vi "VersaLaseGUI_ForMain_v3.vi"() -> ()   [LabVIEW 2014]
uses:
  D:/Box Sync/Res/LabVIEW/Ts LabVIEW Code/avo/VersaUSB/VersaUSB.dll
  VersaUSB.dll
panel:
  out "Grn Temp 2":dbl
  out "ne":i32
  out "e":i32
  in  "Blu Pow":dbl(slide) scale=0.0..100.0
  in  "Grn Pow":dbl(slide) scale=0.0..40.0
  in  "Blu On":bool
  in  "Grn On":bool
  out "Blu Temp":dbl
  out "Grn Temp":dbl
  in  "Red Pow":dbl(slide) scale=0.0..100.0
  in  "Red On":bool
  out "Red Temp":dbl
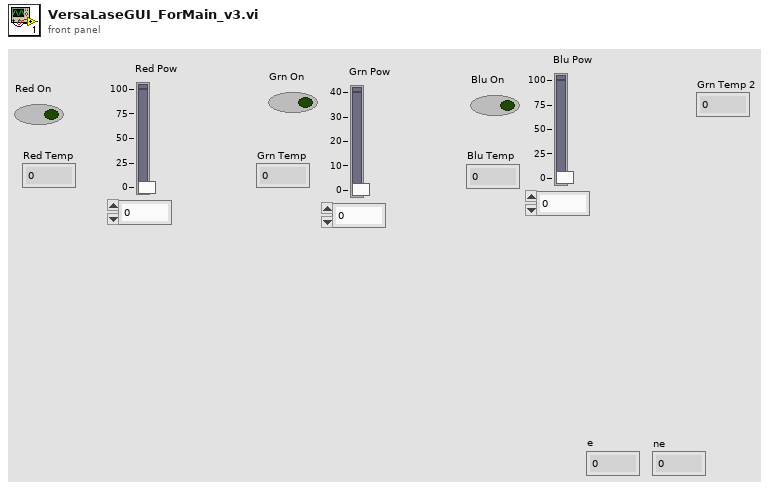
[diagram p1: front panel]
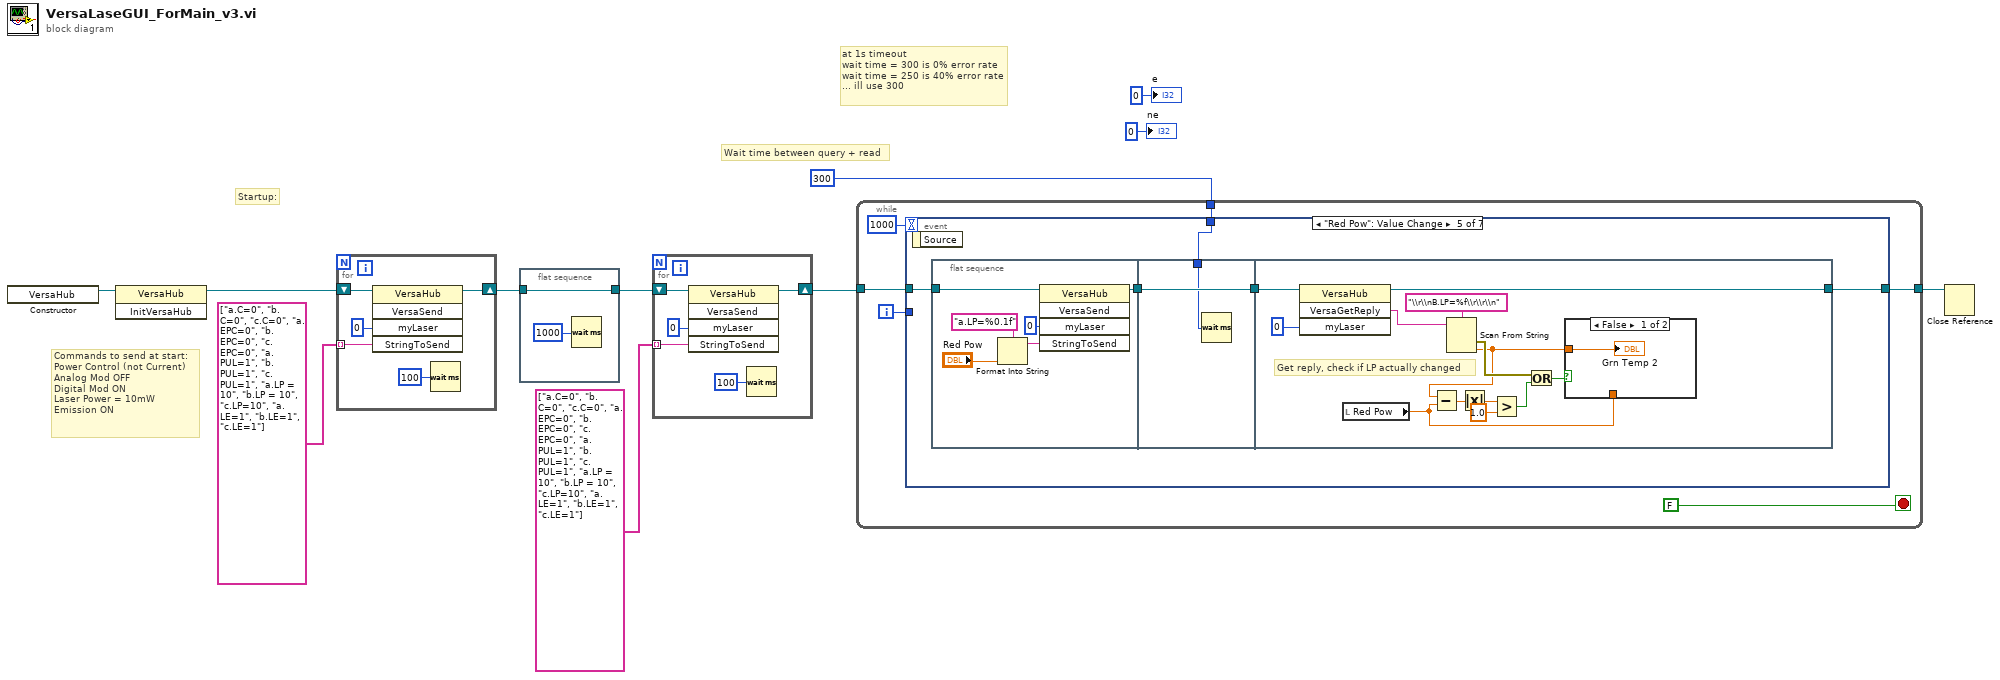
[diagram p0: block diagram]
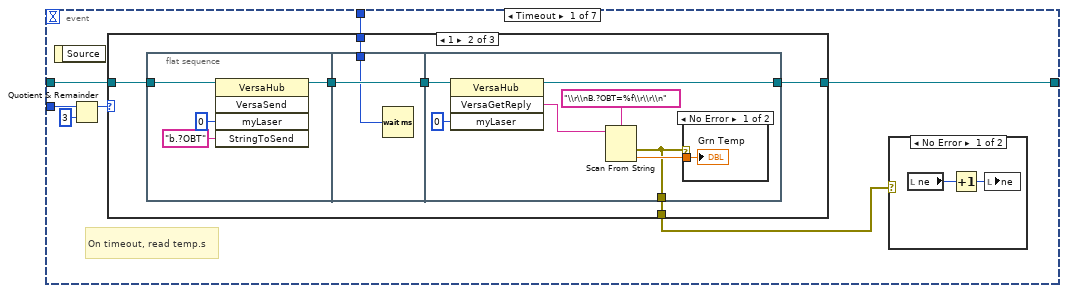
[diagram p2: hidden frame]
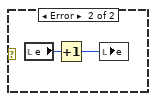
[diagram p3: hidden frame]
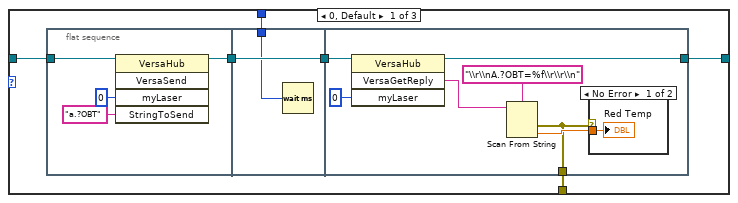
[diagram p4: hidden frame]
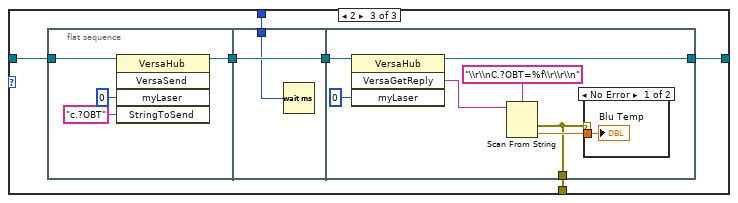
[diagram p7: hidden frame]
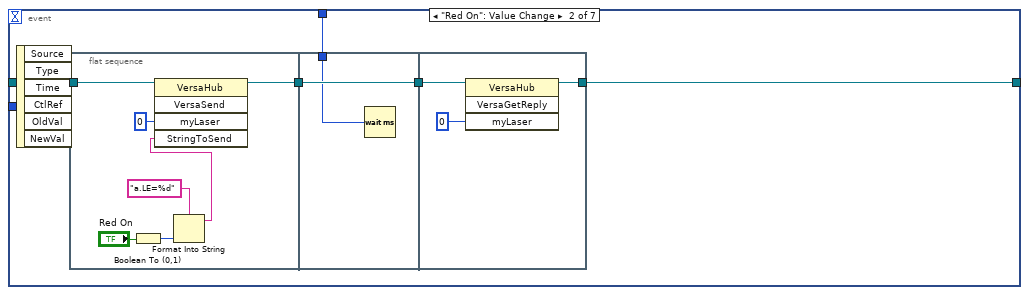
[diagram p9: hidden frame]
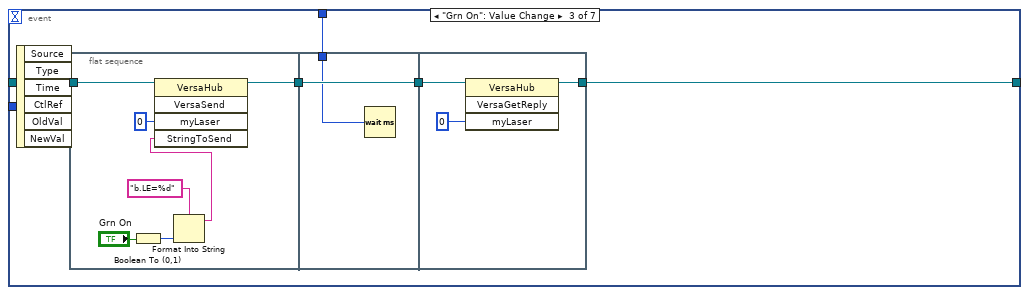
[diagram p10: hidden frame]
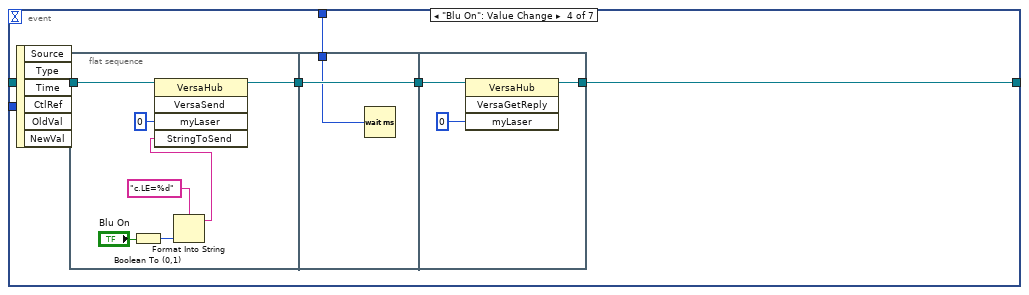
[diagram p11: hidden frame]
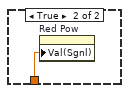
[diagram p12: hidden frame]
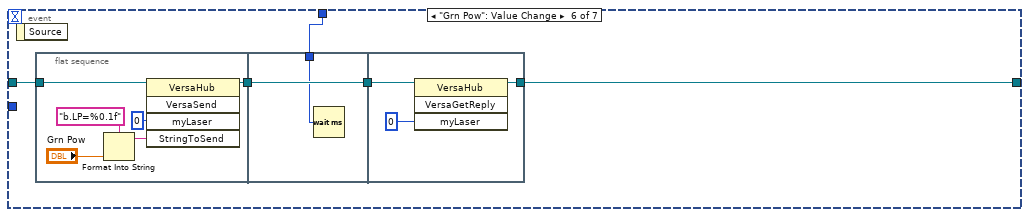
[diagram p13: hidden frame]
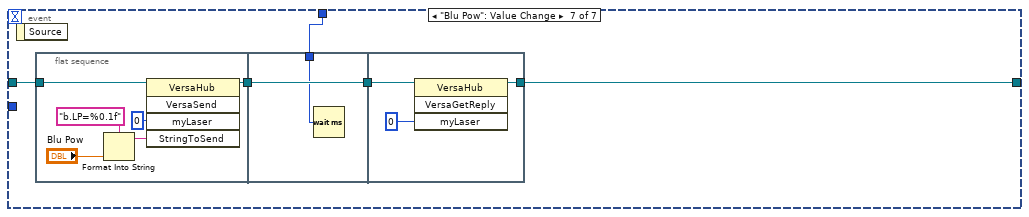
[diagram p14: hidden frame]
diagram:
  # "Startup:"
  # "Wait time between query + read"
  # "Commands to send at start:\nPower Control (not Current)\nAnalog Mod OFF\nDigital Mod ON\nLaser Power = 10mW\nEmission ON"
  # "at 1s timeout\nwait time = 300 is 0% error rate\nwait time = 250 is 40% error rate\n... ill use 300"
  n1 = constructor class="VersaHub"() -> (reference out=w11:refnum<k24>)  [unwired: 3 in, 2 out]
  n2 = invoke class="VersaHub" method="InitVersaHub"(reference=w11) -> (reference out=w5:refnum<k24>)  [unwired: 2 in, 2 out]
  n3 = for {
    tunnel: string[] ["a.C=0", "b.C=0", "c.C=0", "a.EPC=0", "b.EPC=0", "c.EPC=0", "a.PUL=1", "b.PUL=1", "c.PUL=1", "a.LP = 10", "b.LP = 10", "c.LP=10", "a.LE=1", "b.LE=1", "c.LE=1"] -> [w15] mode=indexing
    shift-right: [w14] -> w1
    shift-left: w5 -> [w13]
    n4 = invoke class="VersaHub" method="VersaSend"(reference=w13, "myLaser"=0 ("moduleId"), "StringToSend"=w15) -> (reference out=w14:refnum<k24>)  [unwired: 2 in, 4 out]
    n5 = Wait (ms)(milliseconds to wait=u32 100) -> ()  [unwired: 1 out]
  }
  n6 = flat-sequence {
    tunnel: [w18] -> w2
    tunnel: w1 -> [w18]
    frame #0 {
      n7 = Wait (ms)(milliseconds to wait=u32 1000) -> ()  [unwired: 1 out]
    }
  }
  n8 = for {
    tunnel: string[] ["a.C=0", "b.C=0", "c.C=0", "a.EPC=0", "b.EPC=0", "c.EPC=0", "a.PUL=1", "b.PUL=1", "c.PUL=1", "a.LP = 10", "b.LP = 10", "c.LP=10", "a.LE=1", "b.LE=1", "c.LE=1"] -> [w22] mode=indexing
    shift-right: [w21] -> w3
    shift-left: w2 -> [w20]
    n9 = invoke class="VersaHub" method="VersaSend"(reference=w20, "myLaser"=0 ("moduleId"), "StringToSend"=w22) -> (reference out=w21:refnum<k24>)  [unwired: 2 in, 4 out]
    n10 = Wait (ms)(milliseconds to wait=u32 100) -> ()  [unwired: 1 out]
  }
  n11 = while {
    tunnel: w3 -> [w29]
    tunnel: [w28] -> w10
    tunnel: u32 300 -> [w24]
    i -> [w25]
    stop <- FALSE stop-if-true
    n12 = event shown="[4] \"Red Pow\": Value Change" {
      selector: _ -> [_ _ _ _ _ _ _]
      dyn-events: _ -> [_ _ _ _ _ _ _]
      timeout: 1000 -> [_ _ _ _ _ _ _]
      tunnel: w29 -> [w36 w105 w122 w139 w154 w182 w198]
      tunnel: [w30 w102 w119 w136 w153 w181 w197] -> w28
      tunnel: w25 -> [w35 _ _ _ _ _ _]
      tunnel: w24 -> [w32 w101 w118 w135 w152 w180 w196]
      event Timeout {
        # "On timeout, read temp.s"
        n13 = event-data() -> ()  [unwired: 1 in, 1 out]
        n14 = Quotient & Remainder(x=w35, y=3) -> (x-y*floor(x/y)=w34:i32)  [unwired: 1 out]
        n15 = case shown="1" w34 {
          tunnel: w36 -> [w44 w64 w84]
          tunnel: [w43 w63 w83] -> w30
          tunnel: w32 -> [w42 w62 w82]
          tunnel: [w41 w61 w81] -> w31
          frame 0, Default {
            n16 = flat-sequence {
              tunnel: w44 -> [w50]
              tunnel: [w47] -> w46
              tunnel: w46 -> [w52]
              tunnel: [w52] -> w45
              tunnel: w42 -> [w51]
              tunnel: [w54] -> w43
              tunnel: w45 -> [w58]
              tunnel: [w53] -> w41
              frame #0 {
                n17 = invoke class="VersaHub" method="VersaSend"(reference=w50, "myLaser"=0, "StringToSend"="a.?OBT") -> (reference out=w47:refnum<k24>)  [unwired: 2 in, 4 out]
              }
              frame #1 {
                n18 = Wait (ms)(milliseconds to wait=w51) -> ()  [unwired: 1 out]
              }
              frame #2 {
                n19 = invoke class="VersaHub" method="VersaGetReply"(reference=w58, "myLaser"=0) -> (reference out=w54:refnum<k24>, "VersaGetReply"=w55:string)  [unwired: 2 in, 2 out]
                n20 = Scan From String(format string="\\r\\nA.?OBT=%f\\r\\r\\n", input string=w55) -> (error out=w53:errorcluster, output 1=w56:dbl)  [unwired: 3 in, 2 out]
                n21 = case shown="No Error" w53 {
                  tunnel: w56 -> [w60 _]
                  frame No Error {
                    "Red Temp" <- w60
                  }
                  frame Error {
                  }
                }
              }
            }
          }
          frame 1 {
            n22 = flat-sequence {
              tunnel: w64 -> [w70]
              tunnel: [w67] -> w66
              tunnel: w66 -> [w72]
              tunnel: [w72] -> w65
              tunnel: w62 -> [w71]
              tunnel: [w74] -> w63
              tunnel: w65 -> [w78]
              tunnel: [w73] -> w61
              frame #0 {
                n23 = invoke class="VersaHub" method="VersaSend"(reference=w70, "myLaser"=0, "StringToSend"="b.?OBT") -> (reference out=w67:refnum<k24>)  [unwired: 2 in, 4 out]
              }
              frame #1 {
                n24 = Wait (ms)(milliseconds to wait=w71) -> ()  [unwired: 1 out]
              }
              frame #2 {
                n25 = invoke class="VersaHub" method="VersaGetReply"(reference=w78, "myLaser"=0) -> (reference out=w74:refnum<k24>, "VersaGetReply"=w75:string)  [unwired: 2 in, 2 out]
                n26 = Scan From String(format string="\\r\\nB.?OBT=%f\\r\\r\\n", input string=w75) -> (error out=w73:errorcluster, output 1=w76:dbl)  [unwired: 3 in, 2 out]
                n27 = case shown="No Error" w73 {
                  tunnel: w76 -> [w80 _]
                  frame No Error {
                    "Grn Temp" <- w80
                  }
                  frame Error {
                  }
                }
              }
            }
          }
          frame 2 {
            n28 = flat-sequence {
              tunnel: w84 -> [w90]
              tunnel: [w87] -> w86
              tunnel: w86 -> [w92]
              tunnel: [w92] -> w85
              tunnel: w82 -> [w91]
              tunnel: [w94] -> w83
              tunnel: w85 -> [w98]
              tunnel: [w93] -> w81
              frame #0 {
                n29 = invoke class="VersaHub" method="VersaSend"(reference=w90, "myLaser"=0, "StringToSend"="c.?OBT") -> (reference out=w87:refnum<k24>)  [unwired: 2 in, 4 out]
              }
              frame #1 {
                n30 = Wait (ms)(milliseconds to wait=w91) -> ()  [unwired: 1 out]
              }
              frame #2 {
                n31 = invoke class="VersaHub" method="VersaGetReply"(reference=w98, "myLaser"=0) -> (reference out=w94:refnum<k24>, "VersaGetReply"=w95:string)  [unwired: 2 in, 2 out]
                n32 = Scan From String(format string="\\r\\nC.?OBT=%f\\r\\r\\n", input string=w95) -> (error out=w93:errorcluster, output 1=w96:dbl)  [unwired: 3 in, 2 out]
                n33 = case shown="No Error" w93 {
                  tunnel: w96 -> [w100 _]
                  frame No Error {
                    "Blu Temp" <- w100
                  }
                  frame Error {
                  }
                }
              }
            }
          }
        }
        n34 = case shown="No Error" w31 {
          frame No Error {
            n35 = local read "ne"() -> (w38:i32)
            n36 = Increment(x=w38) -> (x+1=w37:i32)
            n37 = local write "ne"(w37) -> ()
          }
          frame Error {
            n38 = local read "e"() -> (w39:i32)
            n39 = Increment(x=w39) -> (x+1=w40:i32)
            n40 = local write "e"(w40) -> ()
          }
        }
      }
      event "Red On": Value Change {
        n41 = event-data() -> ()  [unwired: 1 in, 6 out]
        n42 = flat-sequence {
          tunnel: w105 -> [w112]
          tunnel: [w110] -> w104
          tunnel: w104 -> [w114]
          tunnel: [w114] -> w103
          tunnel: w101 -> [w113]
          tunnel: [w115] -> w102
          tunnel: w103 -> [w116]
          frame #0 {
            n43 = Boolean To (0,1)(Boolean="Red On") -> (0, 1=w108:i16)
            n44 = Format Into String(format string="a.LE=%d", w108) -> (resulting string=w106:string)  [unwired: 2 in, 1 out]
            n45 = invoke class="VersaHub" method="VersaSend"(reference=w112, "myLaser"=0, "StringToSend"=w106) -> (reference out=w110:refnum<k24>)  [unwired: 2 in, 4 out]
          }
          frame #1 {
            n46 = Wait (ms)(milliseconds to wait=w113) -> ()  [unwired: 1 out]
          }
          frame #2 {
            n47 = invoke class="VersaHub" method="VersaGetReply"(reference=w116, "myLaser"=0) -> (reference out=w115:refnum<k24>)  [unwired: 2 in, 3 out]
          }
        }
      }
      event "Grn On": Value Change {
        n48 = event-data() -> ()  [unwired: 1 in, 6 out]
        n49 = flat-sequence {
          tunnel: w122 -> [w129]
          tunnel: [w127] -> w121
          tunnel: w121 -> [w131]
          tunnel: [w131] -> w120
          tunnel: w118 -> [w130]
          tunnel: [w132] -> w119
          tunnel: w120 -> [w133]
          frame #0 {
            n50 = Boolean To (0,1)(Boolean="Grn On") -> (0, 1=w125:i16)
            n51 = Format Into String(format string="b.LE=%d", w125) -> (resulting string=w123:string)  [unwired: 2 in, 1 out]
            n52 = invoke class="VersaHub" method="VersaSend"(reference=w129, "myLaser"=0, "StringToSend"=w123) -> (reference out=w127:refnum<k24>)  [unwired: 2 in, 4 out]
          }
          frame #1 {
            n53 = Wait (ms)(milliseconds to wait=w130) -> ()  [unwired: 1 out]
          }
          frame #2 {
            n54 = invoke class="VersaHub" method="VersaGetReply"(reference=w133, "myLaser"=0) -> (reference out=w132:refnum<k24>)  [unwired: 2 in, 3 out]
          }
        }
      }
      event "Blu On": Value Change {
        n55 = event-data() -> ()  [unwired: 1 in, 6 out]
        n56 = flat-sequence {
          tunnel: w139 -> [w146]
          tunnel: [w144] -> w138
          tunnel: w138 -> [w148]
          tunnel: [w148] -> w137
          tunnel: w135 -> [w147]
          tunnel: [w149] -> w136
          tunnel: w137 -> [w150]
          frame #0 {
            n57 = Boolean To (0,1)(Boolean="Blu On") -> (0, 1=w142:i16)
            n58 = Format Into String(format string="c.LE=%d", w142) -> (resulting string=w140:string)  [unwired: 2 in, 1 out]
            n59 = invoke class="VersaHub" method="VersaSend"(reference=w146, "myLaser"=0, "StringToSend"=w140) -> (reference out=w144:refnum<k24>)  [unwired: 2 in, 4 out]
          }
          frame #1 {
            n60 = Wait (ms)(milliseconds to wait=w147) -> ()  [unwired: 1 out]
          }
          frame #2 {
            n61 = invoke class="VersaHub" method="VersaGetReply"(reference=w150, "myLaser"=0) -> (reference out=w149:refnum<k24>)  [unwired: 2 in, 3 out]
          }
        }
      }
      event "Red Pow": Value Change {
        n62 = event-data() -> ()  [unwired: 1 in, 1 out]
        n63 = flat-sequence {
          tunnel: w154 -> [w162]
          tunnel: [w160] -> w156
          tunnel: w156 -> [w164]
          tunnel: [w164] -> w155
          tunnel: w152 -> [w163]
          tunnel: [w175] -> w153
          tunnel: w155 -> [w176]
          frame #0 {
            n64 = Format Into String(format string="a.LP=%0.1f", "Red Pow") -> (resulting string=w157:string)  [unwired: 2 in, 1 out]
            n65 = invoke class="VersaHub" method="VersaSend"(reference=w162, "myLaser"=0, "StringToSend"=w157) -> (reference out=w160:refnum<k24>)  [unwired: 2 in, 4 out]
          }
          frame #1 {
            n66 = Wait (ms)(milliseconds to wait=w163) -> ()  [unwired: 1 out]
          }
          frame #2 {
            # "Get reply, check if LP actually changed"
            n67 = invoke class="VersaHub" method="VersaGetReply"(reference=w176, "myLaser"=0) -> (reference out=w175:refnum<k24>, "VersaGetReply"=w173:string)  [unwired: 2 in, 2 out]
            n68 = local read "Red Pow"() -> (w170:dbl)
            n69 = Scan From String(format string="\\r\\nB.LP=%f\\r\\r\\n", input string=w173) -> (error out=w172:errorcluster, output 1=w171:dbl)  [unwired: 3 in, 2 out]
            n70 = Subtract(x=w171, y=w170) -> (x-y=w169:dbl)
            n71 = Absolute Value(x=w169) -> (abs(x)=w167:dbl)
            n72 = Greater?(x=w167, y=1.0) -> (0:w166:bool)
            n73 = Or(x=w172, y=w166) -> (x .or. y?=w168:bool)
            n74 = case shown="False" w168 {
              tunnel: w171 -> [w178 _]
              tunnel: w170 -> [_ w179]
              frame False {
                "Grn Temp 2" <- w178
              }
              frame True {
                n75 = property on="Red Pow" class="Slide (strict)"("Val(Sgnl)"=w179) -> ()  [unwired: 2 in, 2 out]
              }
            }
          }
        }
      }
      event "Grn Pow": Value Change {
        n76 = event-data() -> ()  [unwired: 1 in, 1 out]
        n77 = flat-sequence {
          tunnel: w182 -> [w190]
          tunnel: [w188] -> w184
          tunnel: w184 -> [w192]
          tunnel: [w192] -> w183
          tunnel: w180 -> [w191]
          tunnel: [w193] -> w181
          tunnel: w183 -> [w194]
          frame #0 {
            n78 = Format Into String(format string="b.LP=%0.1f", "Grn Pow") -> (resulting string=w185:string)  [unwired: 2 in, 1 out]
            n79 = invoke class="VersaHub" method="VersaSend"(reference=w190, "myLaser"=0, "StringToSend"=w185) -> (reference out=w188:refnum<k24>)  [unwired: 2 in, 4 out]
          }
          frame #1 {
            n80 = Wait (ms)(milliseconds to wait=w191) -> ()  [unwired: 1 out]
          }
          frame #2 {
            n81 = invoke class="VersaHub" method="VersaGetReply"(reference=w194, "myLaser"=0) -> (reference out=w193:refnum<k24>)  [unwired: 2 in, 3 out]
          }
        }
      }
      event "Blu Pow": Value Change {
        n82 = event-data() -> ()  [unwired: 1 in, 1 out]
        n83 = flat-sequence {
          tunnel: w198 -> [w206]
          tunnel: [w204] -> w200
          tunnel: w200 -> [w208]
          tunnel: [w208] -> w199
          tunnel: w196 -> [w207]
          tunnel: [w209] -> w197
          tunnel: w199 -> [w210]
          frame #0 {
            n84 = Format Into String(format string="b.LP=%0.1f", "Blu Pow") -> (resulting string=w201:string)  [unwired: 2 in, 1 out]
            n85 = invoke class="VersaHub" method="VersaSend"(reference=w206, "myLaser"=0, "StringToSend"=w201) -> (reference out=w204:refnum<k24>)  [unwired: 2 in, 4 out]
          }
          frame #1 {
            n86 = Wait (ms)(milliseconds to wait=w207) -> ()  [unwired: 1 out]
          }
          frame #2 {
            n87 = invoke class="VersaHub" method="VersaGetReply"(reference=w210, "myLaser"=0) -> (reference out=w209:refnum<k24>)  [unwired: 2 in, 3 out]
          }
        }
      }
    }
  }
  n88 = Close Reference(reference=w10) -> ()  [unwired: 1 in, 1 out]
  "e" <- 0 ("e")
  "ne" <- 0 ("ne")
